vi "Autonomous.vi"(11 "Call Context":T7) -> (0 "SubState 2":T2, 1 "Loop 2 Data":T3, 2 "SubState 1":T2, 3 "Loop 1 Data":T4, 4 "Loop 3 Data":T1, 5 "SubState 0":T2=enum."driver control", 6 "SubState 3":T2, 7 "Loop 0 Data":T5, 10 "SubState 4":T6)   [LabVIEW 2013]
uses:
  typedefs/subStates.ctl
  <vilib>/Rock Robotics/WPI/DriverStation/WPI_DriverStationDerivedRobotMode.ctl
  typedefs/singleUseSubstate.ctl
  typedefs/Loop Datatypes/Loop 0 Datatype.ctl
  typedefs/Loop Datatypes/Loop 1 Datatype.ctl
  typedefs/Loop Datatypes/Loop 2 Datatype.ctl
  typedefs/Loop Datatypes/Loop 3 Datatype.ctl
  typedefs/fg_typedef.ctl
  typedefs/vision enable.ctl
panel:
  # "Autonomous Loop Data"
  # "Robot Drive"
  # "State Machine Master"
  # "Pickup/Passing Belts"
  # "Pickup/Passing Arm"
  # "Pneumatics"
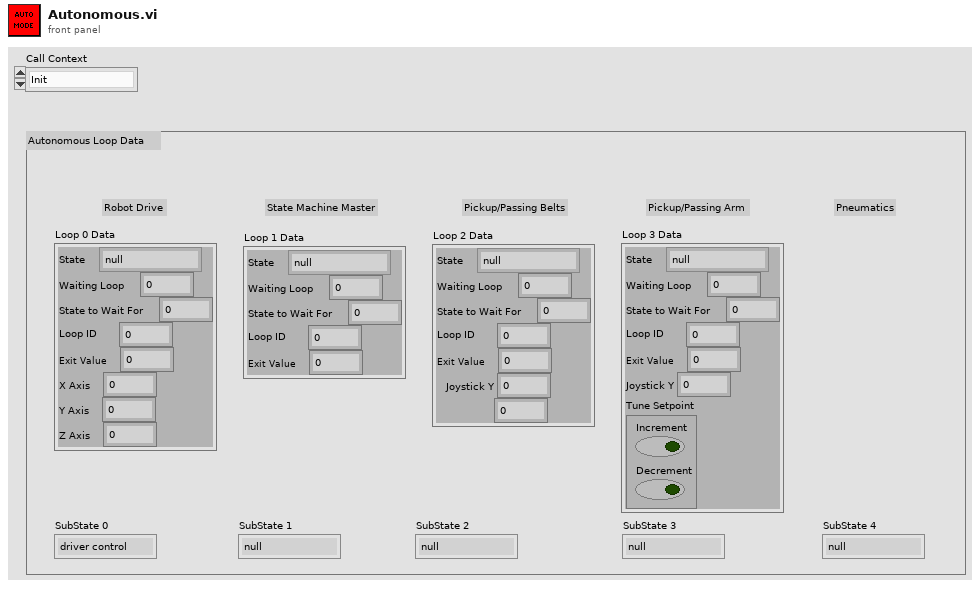
[diagram p1: front panel]
types:
  T1 = typedef "Loop 3 Datatype.ctl" = cluster{"State":T2, "Waiting Loop":i32, "State to Wait For":i32, "Loop ID":i32, "Exit Value":i32, "Joystick Y":dbl, "Tune Setpoint":cluster{"Increment":bool, "Decrement":bool}}
  T2 = typedef "subStates.ctl" = enum16{"null", "wait", "driver control", "auto", "manual override", "hold position", "rotate", "pickup", "pass", "load", "goto shoot", "shoot high goal", "shoot low goal", "cancel arm", "cancel shooter", "end"}
  T3 = typedef "Loop 2 Datatype.ctl" = cluster{"State":T2, "Waiting Loop":i32, "State to Wait For":i32, "Loop ID":i32, "Exit Value":i32, "Joystick Y":dbl, "Joystick Z":dbl}
  T4 = typedef "Loop 1 Datatype.ctl" = cluster{"State":T2, "Waiting Loop":i32, "State to Wait For":i32, "Loop ID":i32, "Exit Value":i32}
  T5 = typedef "Loop 0 Datatype.ctl" = cluster{"State":T2, "Waiting Loop":i32, "State to Wait For":i32, "Loop ID":i32, "Exit Value":i32, "X Axis":dbl, "Y Axis":dbl, "Z Axis":dbl}
  T6 = typedef "singleUseSubstate.ctl" = enum16{"null", "wait", "shift high", "shift low", "extend shooter", "retract shooter", "latch", "unlatch"}
  T7 = typedef "WPI_DriverStationDerivedRobotMode.ctl" = enum16{"Init", "Execute", "Stop"}
  T8 = typedef "vision enable.ctl" = enum16{"Enable", "Disable", "Stop"}
  T9 = typedef "fg_typedef.ctl" = enum16{"Get", "Set"}
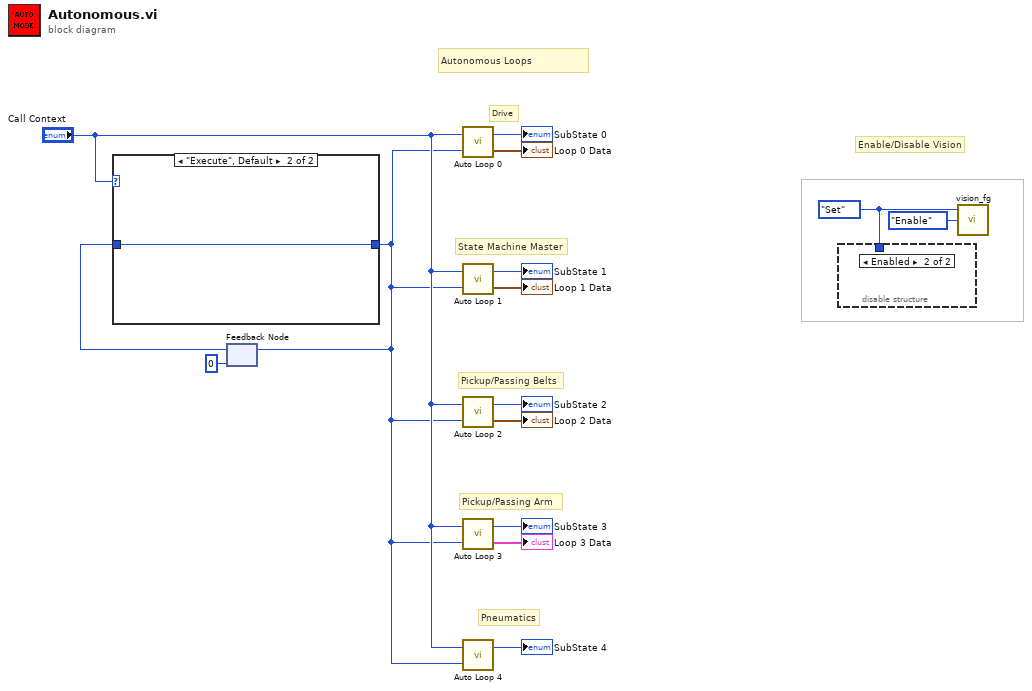
[diagram p0: block diagram]
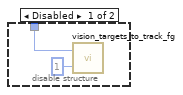
[diagram p2: hidden frame]
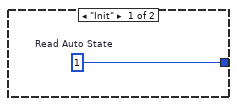
[diagram p3: hidden frame]
diagram:
  w2 = fg_typedef."Set" ("Menu")
  # "Autonomous Loops"
  # "Enable/Disable Vision"
  # "Pickup/Passing Arm"
  # "Pickup/Passing Belts"
  # "Pneumatics"
  # "State Machine Master"
  # "Drive"
  n1 = feedback #1(u8 0 ("Read Auto State")) -> (w3:u8)
  n2 = case shown="\"Execute\", Default" "Call Context" {
    tunnel: [w16 w17] -> w5
    tunnel: w3 -> [_ w17]
    frame "Init" {
      w16 = u8 1  # Read Auto State
    }
    frame "Execute", Default {
    }
  }
  n3 = feedback-in #1(w5) -> ()
  n4 = call "Auto Loop 0.vi"("Auto State"=w5, "Call Context"="Call Context") -> ("Loop 0 Data"=→"Loop 0 Data":T5, "SubState 0"=→"SubState 0":T2)
  n5 = call "Auto Loop 1.vi"("Auto State"=w5, "Call Context"="Call Context") -> ("Loop 1 Data"=→"Loop 1 Data":T4, "SubState 1"=→"SubState 1":T2)
  n6 = call "Auto Loop 2.vi"("Auto State"=w5, "Call Context"="Call Context") -> ("Loop 2 Data"=→"Loop 2 Data":T3, "SubState 2"=→"SubState 2":T2)
  n7 = call "Auto Loop 3.vi"("Auto State"=w5, "Call Context"="Call Context") -> ("Loop 3 Data"=→"Loop 3 Data":T1, "SubState 3"=→"SubState 3":T2)
  n8 = call "Auto Loop 4.vi"("Auto State"=w5, "Call Context"="Call Context") -> ("SubState 5"=→"SubState 4":T6)  [unwired: 1 in]
  n9 = disable-structure shown="Enabled" {
    disable-tunnel: w2 -> [w19 _]
    frame Disabled {
      n10 = call "vision_targets_to_track_fg.vi"("Input"=1, "Menu (Get)"=w19) -> ()  [unwired: 1 out]
    }
    frame Enabled {
    }
  }
  n11 = call "vision_fg.vi"("Action"=vision_enable."Enable", "Menu"=w2) -> ()  [unwired: 1 in, 2 out]
